vi "Get Remaining Timeout.vi"(0 "timeout (100 ms)":dbl, 5 "start time":timestamp, 11 "error in":errorcluster) -> (4 "remaining timeout":dbl, 6 "timed out?":bool, 15 "error out":errorcluster)   [LabVIEW 2014, in "niHighSpeedSerial Eye Scan Common v1 Host.lvlib"]
doc: "Returns the amount of time remaining given the <b>start time</b>.\nIf the timeout has been reached, <b>timed out</b> will be set to true.\n\n<B>Input Parameters</B>\n\n<B>timeout (100 ms)</B> The amount of time (in seconds) before timing timing out.\nSpecifying '-1' prevents 'timed out' from ever returning true.\n\n<B>start time</B> The time to compare against the current time to see if the timeout has been reached.\n\n<B>error in</B> describes error conditions that occur before this node runs. This input provides standard 'error in' functionality.\n\n<B>Output Parameters</B>\n\n<B>remaining timeout</B> The amount of time remaining before timeout occurs. If timeout occurs, this value will be '0'.\n\n<B>timed out?</B> returns true if at least 'timeout' amount of time has passed.\n\n<B>error out</B> contains error information. This output provides standard 'error out' functionality."
uses:
  <instrlib>/niHighSpeedSerial/Eye Scan/v1/Host/Common/niHighSpeedSerial Eye Scan Common v1 Host.lvlib
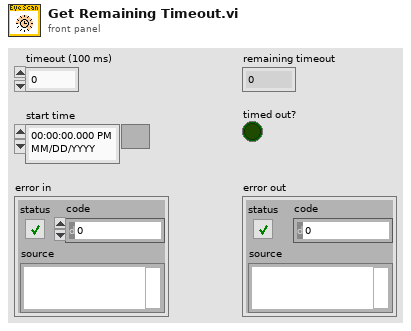
[diagram p1: front panel]
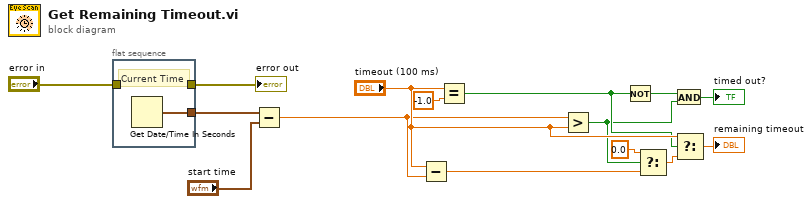
[diagram p0: block diagram]
diagram:
  n1 = flat-sequence {
    tunnel: "error in" -> [w17]
    tunnel: [w17] -> w12
    tunnel: [w16] -> w13
    frame #0 {
      # "Current Time"
      n2 = Get Date/Time In Seconds() -> (seconds since 1Jan1904=w16:timestamp)
    }
  }
  n3 = Subtract(x=w13, y="start time") -> (x-y=w6:dbl)
  n4 = Subtract(x="timeout (100 ms)", y=w6) -> (x-y=w5:dbl)
  n5 = Equal?(x="timeout (100 ms)", y=-1.0) -> (x = y?=w4:bool)
  n6 = Greater?(x=w6, y="timeout (100 ms)") -> (0:w3:bool)
  n7 = Not(x=w4) -> (.not. x?=w2:bool)
  n8 = Select(t=0.0, s=w3, f=w5) -> (s? t:f=w7:dbl)
  n9 = And(x=w2, y=w3) -> (x .and. y?=→"timed out?":bool)
  n10 = Select(t="timeout (100 ms)", s=w4, f=w7) -> (s? t:f=→"remaining timeout":dbl)
  "error out" <- w12
